vi "Translator.GatherControlsByRef.vi"(8 "error in":errorcluster, 11 "Front Panel":refnum<vi>) -> (0 "error out":errorcluster, 2 "Controls out":T1[](array[typedef]))   [LabVIEW 2016]
uses:
  Translator.ControlData.ctl
  Translator.ControlTypes.ctl
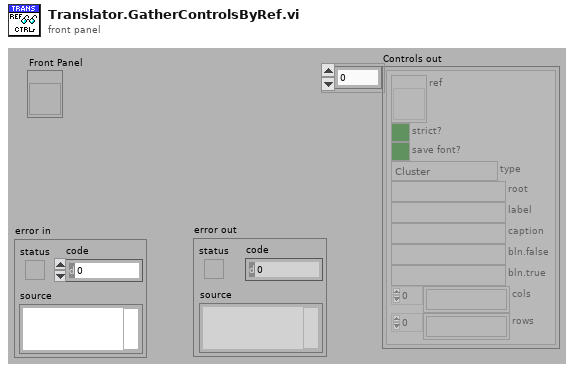
[diagram p1: front panel]
types:
  T1 = typedef "Translator.ControlData.ctl" = cluster{"ref":refnum<vi>, "strict?":bool, "save font?":bool, "type":T2, "root":string, "label":string, "caption":string, "bln.false":string, "bln.true":string, "cols":string[], "rows":string[]}
  T2 = typedef "Translator.ControlTypes.ctl" = enum16{"Cluster", "Array", "Boolean", "Ring", "String", "Tab", "Listbox", "Multicolumn listbox", "Table", "Tree", "Other"}
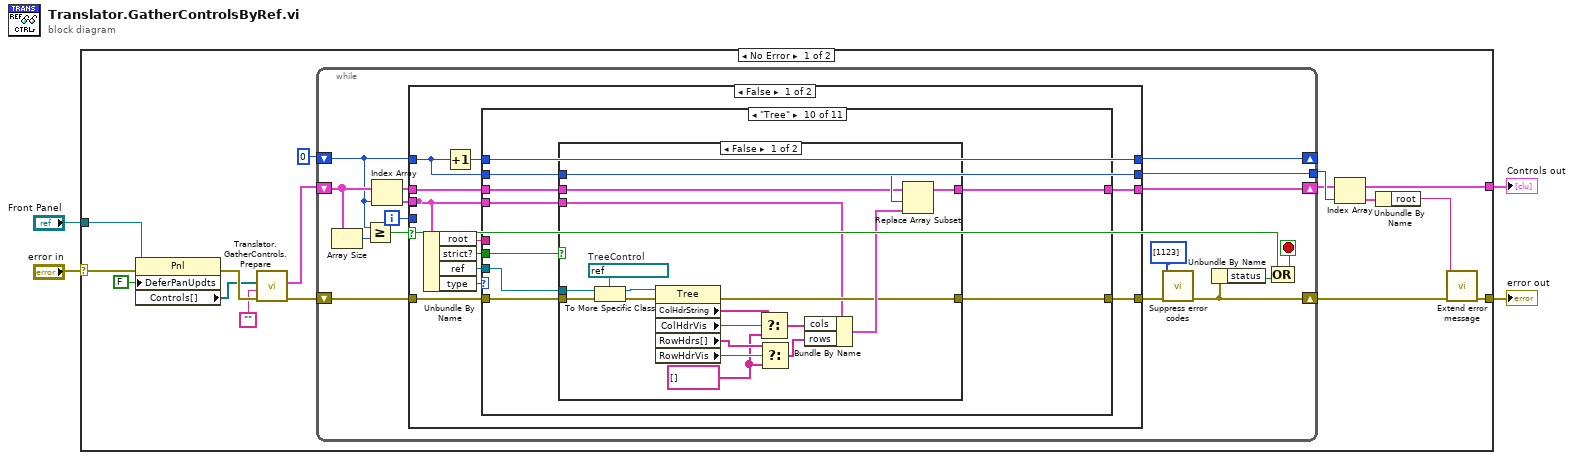
[diagram p0: block diagram]
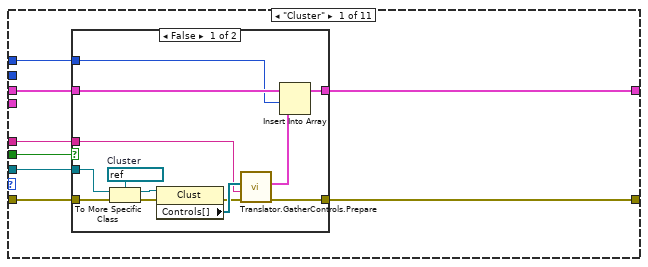
[diagram p2: hidden frame]
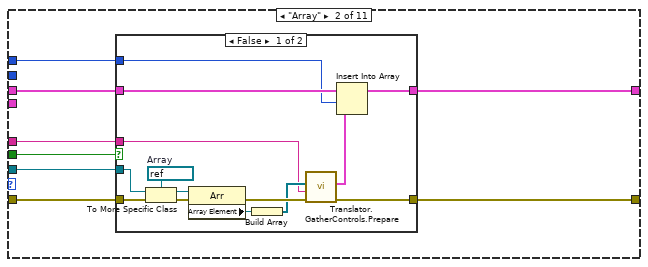
[diagram p4: hidden frame]
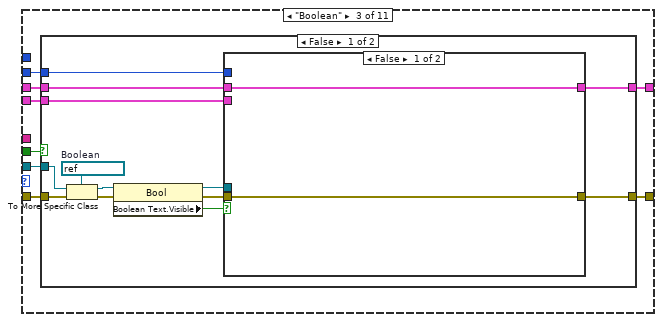
[diagram p6: hidden frame]
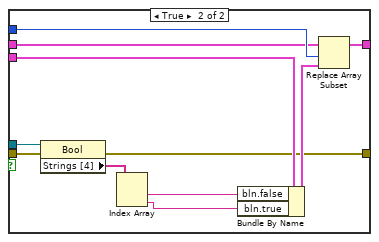
[diagram p7: hidden frame]
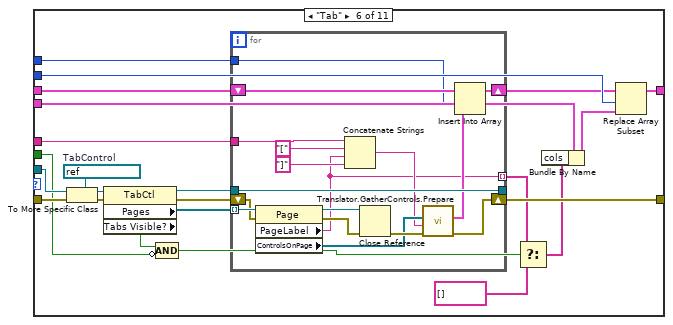
[diagram p11: hidden frame]
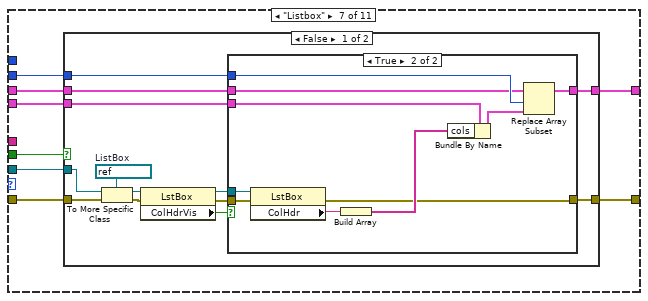
[diagram p12: hidden frame]
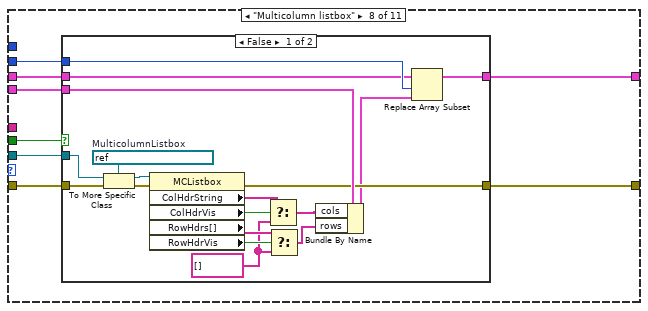
[diagram p15: hidden frame]
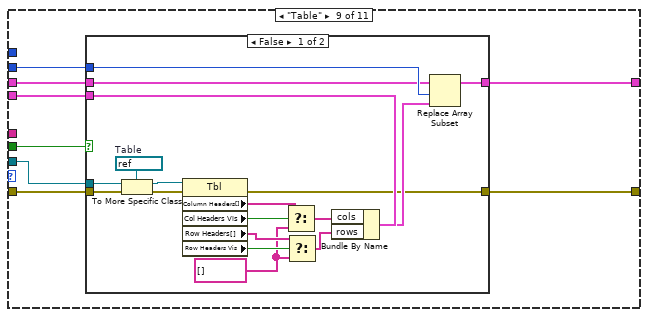
[diagram p17: hidden frame]
diagram:
  n1 = case shown="No Error" "error in" {
    selector: "error in" -> [w7 w297]
    tunnel: [w14 w297] -> w3
    tunnel: [w10 _] -> w2
    tunnel: "Front Panel" -> [w6 _]
    frame No Error {
      n2 = property class="Pnl"(reference=w6, error in=w7, "DeferPanUpdts"=FALSE ("Defer Panel Updates")) -> (error out=w17:errorcluster, "Controls[]"=w11:refnum<vi>[])  [unwired: 1 out]
      n3 = call "Translator.GatherControls.Prepare.vi"("error in"=w17, "root"="", "Controls in"=w11) -> ("error out"=w16:errorcluster, "Controls out"=w18:T1[])  [unwired: 7 in]
      n4 = while {
        shift-right: [w30] -> w10
        shift-left: w18 -> [w31]
        shift-right: [w27] -> _
        shift-left: 0 -> [w29]
        tunnel: [w28] -> w12
        shift-right: [w23] -> w5
        shift-left: w16 -> [w32]
        i -> [w20]
        stop <- w24 stop-if-true
        n5 = Array Size(array=w31) -> (size(s)=w34:i32)
        n6 = Greater Or Equal?(x=w29, y=w34) -> (x >= y?=w25:bool)
        n7 = Index Array(array=w31, index=w29) -> (element=w21:T1)
        n8 = case shown="False" w25 {
          tunnel: w21 -> [w36 _]
          tunnel: w32 -> [w43 w295]
          tunnel: w31 -> [w42 w296]
          tunnel: w29 -> [w37 w294]
          tunnel: [w35 w296] -> w30
          tunnel: [w41 w295] -> w26
          tunnel: [w37 w294] -> w28
          tunnel: [w40 w294] -> w27
          tunnel: w21 -> [_ _]
          tunnel: w20 -> [_ _]
          frame False {
            n9 = Unbundle By Name(w36) -> ("root"=w38:string, "strict?"=w39:bool, "ref"=w44:refnum<vi>, "type"=w45:T2)
            n10 = Increment(x=w37) -> (x+1=w40:i32)
            n11 = case shown="\"Tree\"" w45 {
              tunnel: w44 -> [w53 w76 w99 _ _ w149 w179 w214 w242 w270 _]
              tunnel: w43 -> [w52 w75 w100 w129 w131 w150 w180 w215 w243 w271 w292]
              tunnel: w42 -> [w51 w74 w96 w130 w132 w148 w175 w210 w238 w266 w293]
              tunnel: w40 -> [w50 w73 _ _ _ w147 _ _ _ _ _]
              tunnel: w39 -> [w46 w69 w93 _ _ w137 w173 w208 w236 w264 _]
              tunnel: w36 -> [_ _ w98 _ _ w146 w178 w213 w241 w269 _]
              tunnel: w37 -> [_ _ w97 _ _ w145 w177 w212 w240 w268 _]
              tunnel: [w49 w72 w95 w130 w132 w142 w176 w211 w239 w267 w293] -> w35
              tunnel: [w48 w71 w94 w129 w131 w141 w174 w209 w237 w265 w292] -> w41
              tunnel: w38 -> [w47 w70 _ _ _ w140 _ _ _ _ _]
              frame "Cluster" {
                n12 = case shown="False" w46 {
                  tunnel: w53 -> [w65 _]
                  tunnel: [w56 w68] -> w48
                  tunnel: w52 -> [w62 w68]
                  tunnel: w51 -> [w61 w67]
                  tunnel: [w59 w67] -> w49
                  tunnel: w50 -> [w55 _]
                  tunnel: w47 -> [w54 _]
                  frame False {
                    w66 = refnum<vi> refnum  # Cluster
                    n13 = To More Specific Class(target class=w66, reference=w65, error in=w62) -> (specific class reference=w64:refnum<vi>, error out=w63:errorcluster)
                    n14 = property class="Clust"(reference=w64, error in=w63) -> (error out=w57:errorcluster, "Controls[]"=w60:refnum<vi>[])  [unwired: 1 out]
                    n15 = call "Translator.GatherControls.Prepare.vi"("error in"=w57, "root"=w54, "Controls in"=w60) -> ("error out"=w56:errorcluster, "Controls out"=w58:T1[])  [unwired: 7 in]
                    n16 = Insert Into Array(array=w61, index=w55, new element=w58) -> (w59:T1[])
                  }
                  frame True {
                  }
                }
              }
              frame "Array" {
                n17 = case shown="False" w69 {
                  tunnel: w76 -> [w90 _]
                  tunnel: [w81 w92] -> w71
                  tunnel: w75 -> [w87 w92]
                  tunnel: w74 -> [w86 w91]
                  tunnel: [w84 w91] -> w72
                  tunnel: w73 -> [w80 _]
                  tunnel: w70 -> [w77 _]
                  frame False {
                    w79 = refnum<vi> refnum  # Array
                    n18 = To More Specific Class(target class=w79, reference=w90, error in=w87) -> (specific class reference=w89:refnum<vi>, error out=w88:errorcluster)
                    n19 = property class="Arr"(reference=w89, error in=w88) -> (error out=w82:errorcluster, "Array Element"=w85:refnum<vi>)  [unwired: 1 out]
                    n20 = Build Array(w85) -> (w78:refnum<vi>[])
                    n21 = call "Translator.GatherControls.Prepare.vi"("error in"=w82, "root"=w77, "Controls in"=w78) -> ("error out"=w81:errorcluster, "Controls out"=w83:T1[])  [unwired: 7 in]
                    n22 = Insert Into Array(array=w86, index=w80, new element=w83) -> (w84:T1[])
                  }
                  frame True {
                  }
                }
              }
              frame "Boolean" {
                n23 = case shown="False" w93 {
                  tunnel: w100 -> [w110 w127]
                  tunnel: w99 -> [w109 _]
                  tunnel: w98 -> [w108 _]
                  tunnel: w97 -> [w107 _]
                  tunnel: w96 -> [w106 w128]
                  tunnel: [w105 w128] -> w95
                  tunnel: [w101 w127] -> w94
                  frame False {
                    w113 = refnum<vi> refnum  # Boolean
                    n24 = To More Specific Class(target class=w113, reference=w109, error in=w110) -> (specific class reference=w112:refnum<vi>, error out=w111:errorcluster)
                    n25 = property class="Bool"(reference=w112, error in=w111) -> (reference out=w102:refnum<vi>, error out=w103:errorcluster, "Boolean Text.Visible"=w104:bool)
                    n26 = case shown="False" w104 {
                      tunnel: w108 -> [_ w126]
                      tunnel: w107 -> [_ w122]
                      tunnel: w106 -> [w115 w121]
                      tunnel: [w115 w120] -> w105
                      tunnel: w103 -> [w114 w119]
                      tunnel: w102 -> [_ w118]
                      tunnel: [w114 w117] -> w101
                      frame False {
                      }
                      frame True {
                        n27 = property class="Bool"(reference=w118, error in=w119) -> (error out=w117:errorcluster, "Strings [4]"=w116:string[])  [unwired: 1 out]
                        n28 = Index Array(array=w116) -> (element #1=w125:string, element #2=w124:string)  [unwired: 2 in]
                        n29 = Bundle By Name(cluster=w126, "bln.false"=w125, "bln.true"=w124) -> (w123:T1)
                        n30 = Replace Array Subset(array=w121, new element=w123, index=w122) -> (w120:T1[])
                      }
                    }
                  }
                  frame True {
                  }
                }
              }
              frame "String" {
              }
              frame "Ring" {
              }
              frame "Tab" {
                w155 = refnum<vi> refnum  # TabControl
                n31 = To More Specific Class(target class=w155, reference=w149, error in=w150) -> (specific class reference=w151:refnum<vi>, error out=w154:errorcluster)
                n32 = property class="TabCtl"(reference=w151, error in=w154) -> (reference out=w152:refnum<vi>, error out=w153:errorcluster, "Pages"=w133:refnum<vi>[], "Tabs Visible?"=w136:bool)
                n33 = Compound Arithmetic op=AND(w136, invert w137) -> (w135:bool)
                n34 = for {
                  tunnel: w133 -> [w171] mode=indexing
                  tunnel: w152 -> [w172]
                  tunnel: [w172] -> _
                  shift-right: [w161] -> w141
                  shift-left: w153 -> [w170]
                  shift-right: [w163] -> w144
                  shift-left: w148 -> [w165]
                  tunnel: w147 -> [w162]
                  tunnel: [w156] -> w139 mode=indexing
                  tunnel: w140 -> [w160]
                  n35 = property class="Page"(reference=w171, error in=w170) -> (reference out=w168:refnum<vi>, error out=w169:errorcluster, "PageLabel"=w156:string, "ControlsOnPage"=w166:refnum<vi>[])
                  n36 = Concatenate Strings(w160, "[" ("string"), w156, "]" ("string")) -> (w157:string)
                  n37 = Close Reference(reference=w168, error in (no error)=w169) -> (error out=w167:errorcluster)
                  n38 = call "Translator.GatherControls.Prepare.vi"("error in"=w167, "root"=w157, "Controls in"=w166) -> ("error out"=w161:errorcluster, "Controls out"=w164:T1[])  [unwired: 7 in]
                  n39 = Insert Into Array(array=w165, index=w162, new element=w164) -> (w163:T1[])
                }
                n40 = Select(t=w139, s=w135, f=string[] [] ("pages/legend")) -> (s? t:f=w138:string[])
                n41 = Bundle By Name(cluster=w146, "cols"=w138) -> (w143:T1)
                n42 = Replace Array Subset(array=w144, new element=w143, index=w145) -> (w142:T1[])
              }
              frame "Listbox" {
                n43 = case shown="False" w173 {
                  tunnel: w180 -> [w190 w207]
                  tunnel: w179 -> [w189 _]
                  tunnel: w178 -> [w188 _]
                  tunnel: w177 -> [w187 _]
                  tunnel: [w186 w206] -> w176
                  tunnel: w175 -> [w185 w206]
                  tunnel: [w182 w207] -> w174
                  frame False {
                    w193 = refnum<vi> refnum  # ListBox
                    n44 = To More Specific Class(target class=w193, reference=w189, error in=w190) -> (specific class reference=w191:refnum<vi>, error out=w192:errorcluster)
                    n45 = property class="LstBox"(reference=w191, error in=w192) -> (reference out=w183:refnum<vi>, error out=w181:errorcluster, "ColHdrVis"=w184:bool)
                    n46 = case shown="True" w184 {
                      tunnel: w188 -> [_ w202]
                      tunnel: w187 -> [_ w205]
                      tunnel: [w194 w204] -> w186
                      tunnel: w185 -> [w194 w203]
                      tunnel: w181 -> [w195 w199]
                      tunnel: w183 -> [_ w198]
                      tunnel: [w195 w196] -> w182
                      frame False {
                      }
                      frame True {
                        n47 = property class="LstBox"(reference=w198, error in=w199) -> (error out=w196:errorcluster, "ColHdr"=w200:string)  [unwired: 1 out]
                        n48 = Build Array(w200) -> (w197:string[])
                        n49 = Bundle By Name(cluster=w202, "cols"=w197) -> (w201:T1)
                        n50 = Replace Array Subset(array=w203, new element=w201, index=w205) -> (w204:T1[])
                      }
                    }
                  }
                  frame True {
                  }
                }
              }
              frame "Multicolumn listbox" {
                n51 = case shown="False" w208 {
                  tunnel: w215 -> [w230 w234]
                  tunnel: w214 -> [w229 _]
                  tunnel: w213 -> [w228 _]
                  tunnel: w212 -> [w227 _]
                  tunnel: [w226 w235] -> w211
                  tunnel: w210 -> [w224 w235]
                  tunnel: [w223 w234] -> w209
                  frame False {
                    w219 = string[] [] ("f")
                    w233 = refnum<vi> refnum  # MulticolumnListbox
                    n52 = To More Specific Class(target class=w233, reference=w229, error in=w230) -> (specific class reference=w231:refnum<vi>, error out=w232:errorcluster)
                    n53 = property class="MCListbox"(reference=w231, error in=w232) -> (error out=w223:errorcluster, "ColHdrString"=w222:string[], "ColHdrVis"=w225:bool, "RowHdrs[]"=w220:string[], "RowHdrVis"=w221:bool)  [unwired: 1 out]
                    n54 = Select(t=w222, s=w225, f=w219) -> (s? t:f=w218:string[])
                    n55 = Select(t=w220, s=w221, f=w219) -> (s? t:f=w217:string[])
                    n56 = Bundle By Name(cluster=w228, "cols"=w218, "rows"=w217) -> (w216:T1)
                    n57 = Replace Array Subset(array=w224, new element=w216, index=w227) -> (w226:T1[])
                  }
                  frame True {
                  }
                }
              }
              frame "Table" {
                n58 = case shown="False" w236 {
                  tunnel: w243 -> [w258 w262]
                  tunnel: w242 -> [w257 _]
                  tunnel: w241 -> [w256 _]
                  tunnel: w240 -> [w255 _]
                  tunnel: [w253 w263] -> w239
                  tunnel: w238 -> [w251 w263]
                  tunnel: [w250 w262] -> w237
                  frame False {
                    w246 = string[] [] ("f")
                    w261 = refnum<vi> refnum  # Table
                    n59 = To More Specific Class(target class=w261, reference=w257, error in=w258) -> (specific class reference=w259:refnum<vi>, error out=w260:errorcluster)
                    n60 = property class="Tbl"(reference=w259, error in=w260) -> (error out=w250:errorcluster, "Column Headers[]"=w249:string[], "Col Headers Vis"=w252:bool, "Row Headers[]"=w247:string[], "Row Headers Vis"=w248:bool)  [unwired: 1 out]
                    n61 = Select(t=w249, s=w252, f=w246) -> (s? t:f=w245:string[])
                    n62 = Select(t=w247, s=w248, f=w246) -> (s? t:f=w244:string[])
                    n63 = Bundle By Name(cluster=w256, "cols"=w245, "rows"=w244) -> (w254:T1)
                    n64 = Replace Array Subset(array=w251, new element=w254, index=w255) -> (w253:T1[])
                  }
                  frame True {
                  }
                }
              }
              frame "Tree" {
                n65 = case shown="False" w264 {
                  tunnel: w271 -> [w286 w290]
                  tunnel: w270 -> [w285 _]
                  tunnel: w269 -> [w272 _]
                  tunnel: w268 -> [w284 _]
                  tunnel: [w282 w291] -> w267
                  tunnel: w266 -> [w280 w291]
                  tunnel: [w279 w290] -> w265
                  frame False {
                    w275 = string[] [] ("f")
                    w289 = refnum<vi> refnum  # TreeControl
                    n66 = To More Specific Class(target class=w289, reference=w285, error in=w286) -> (specific class reference=w287:refnum<vi>, error out=w288:errorcluster)
                    n67 = property class="Tree"(reference=w287, error in=w288) -> (error out=w279:errorcluster, "ColHdrString"=w278:string[], "ColHdrVis"=w281:bool, "RowHdrs[]"=w276:string[], "RowHdrVis"=w277:bool)  [unwired: 1 out]
                    n68 = Select(t=w278, s=w281, f=w275) -> (s? t:f=w274:string[])
                    n69 = Select(t=w276, s=w277, f=w275) -> (s? t:f=w273:string[])
                    n70 = Bundle By Name(cluster=w272, "cols"=w274, "rows"=w273) -> (w283:T1)
                    n71 = Replace Array Subset(array=w280, new element=w283, index=w284) -> (w282:T1[])
                  }
                  frame True {
                  }
                }
              }
              frame "Other" {
              }
            }
          }
          frame True {
          }
        }
        n72 = call "Suppress error codes.vi"("error in (no error)"=w26, "suppress codes([43])"=i32[] [1123]) -> ("error out"=w23:errorcluster)  [unwired: 8 in, 1 out]
        n73 = Unbundle By Name(w23) -> ("status"=w33:bool)
        n74 = Compound Arithmetic op=OR(w25, w33) -> (w24:bool)
      }
      n75 = Index Array(array=w10, index=w12) -> (element=w13:T1)
      n76 = Unbundle By Name(w13) -> ("root"=w9:string)
      n77 = call "Extend error message.vi"("error in"=w5, "extra message part"=w9) -> ("error out"=w14:errorcluster)  [unwired: 9 in]
    }
    frame Error {
    }
  }
  "error out" <- w3
  "Controls out" <- w2
